vi "_TEST_ObjCacher5.vi"() -> ()   [LabVIEW 2017]
uses:
  60e1d46a-1f8f-4a80-a672-883c4a1fd00c.vi
  460dbc62-fbc1-44eb-87a7-bfcd0649ced0.vi
  02fa2a04-6ce5-4cab-9284-be115f328e34.vi
  Data/_support/Get DataType Description String.vi
panel:
  out "x-y":u32
  out "String 3":string
  out "String 2":string
  out "String":string
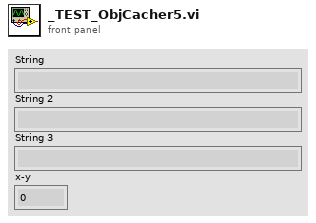
[diagram p1: front panel]
types:
  T1 = cluster{"source":string, "code":i32, "status":bool, "source 2":string}
  T2 = cluster{"source":string, "code":i32, "status":bool, "status 2":bool}
  T3 = cluster{"source":string, "code":i32, "status":bool}
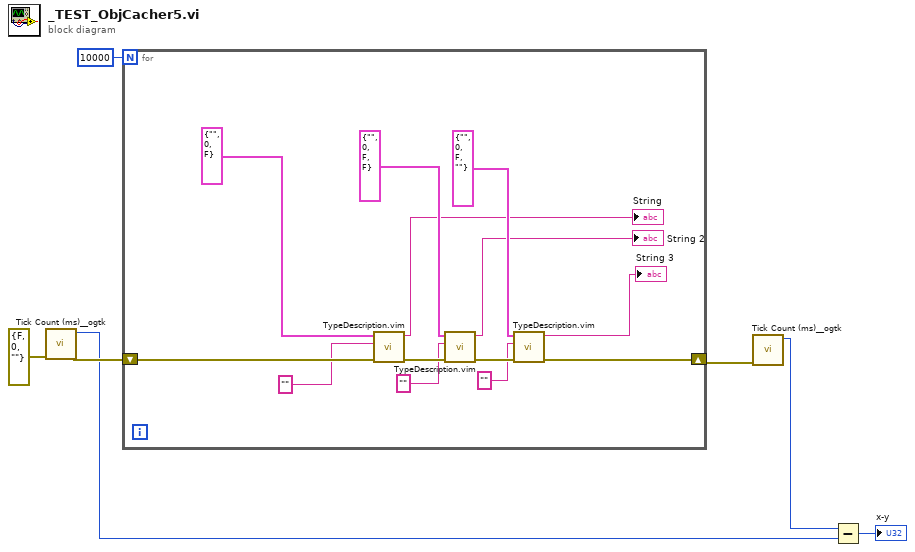
[diagram p0: block diagram]
diagram:
  n1 = call <userlib>:"Tick Count (ms)__ogtk.vi"("error in (no error)"=errorcluster {"status"=FALSE, "code"=0, "source"=""} ("error out")) -> ("error out"=w5:errorcluster, "millisecond timer value"=w2:u32)  [unwired: 9 in]
  n2 = for {
    N: 10000 -> [_]
    shift-right: [w11] -> w4
    shift-left: w5 -> [w12]
    n3 = call "TypeDescription.vim"("error in"=w12, "typeKey(\"\" to use DataTypeDescription)"="" ("typeKey(\"\" to use DataTypeDescription)"), "type"=T3 {"source"="", "code"=0, "status"=FALSE}) -> ("error out"=w18:errorcluster, "String"=→"String":string)  [unwired: 7 in]
    n4 = call "TypeDescription.vim"("error in"=w18, "typeKey(\"\" to use DataTypeDescription)"="" ("typeKey(\"\" to use DataTypeDescription)"), "type"=T2 {"source"="", "code"=0, "status"=FALSE, "status 2"=FALSE}) -> ("error out"=w16:errorcluster, "String"=→"String 2":string)  [unwired: 7 in]
    n5 = call "TypeDescription.vim"("error in"=w16, "typeKey(\"\" to use DataTypeDescription)"="" ("typeKey(\"\" to use DataTypeDescription)"), "type"=T1 {"source"="", "code"=0, "status"=FALSE, "source 2"=""}) -> ("error out"=w11:errorcluster, "String"=→"String 3":string)  [unwired: 7 in]
  }
  n6 = call <userlib>:"Tick Count (ms)__ogtk.vi"("error in (no error)"=w4) -> ("millisecond timer value"=w3:u32)  [unwired: 9 in, 1 out]
  n7 = Subtract(x=w3, y=w2) -> (x-y=→"x-y":u32)
